vi "Check UID Already Exists.vi"(9 "UID":string, 10 "Actor":refnum<class "Actor.lvclass">) -> (2 "Error":errorcluster)   [LabVIEW 2025, in "jettl.lvlib"]
uses:
  jettl.lvlib
  Actor/Actor.lvclass
  Error/Error.lvlib
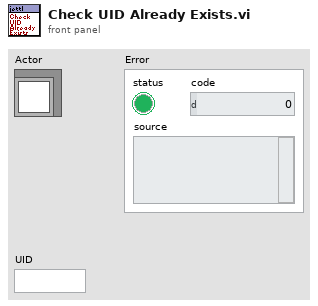
[diagram p1: front panel]
types:
  T1 = typedef "jettl.lvlib/Child UIDs.ctl" = set{string}
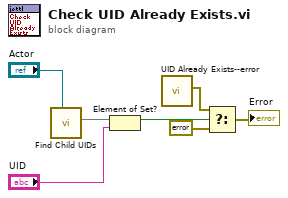
[diagram p0: block diagram]
diagram:
  n1 = call "Find Child UIDs.vi"("Actor in"="Actor") -> ("Child UIDs"=w3:T1)  [unwired: 10 in]
  n2 = Element of Set?(10:"UID", 11:w3) -> (3:w6:bool)
  n3 = call "UID Already Exists--error.vi"() -> ("Error"=w7:errorcluster)  [unwired: 11 in]
  n4 = Select(t=w7, s=w6, f=errorcluster {"status"=FALSE, "code"=0, "source"=""}) -> (s? t:f=→"Error":errorcluster)
